vi "Initialize Menus.vi"(8 "Error In":errorcluster, 11 "Menu Controls":refnum<vi>[](array[refnum])) -> (0 "Error Out":errorcluster)   [LabVIEW 2019, in "LMH-LINX.lvlib"]
uses:
  <vilib>/MakerHub/LINX/LMH-LINX.lvlib
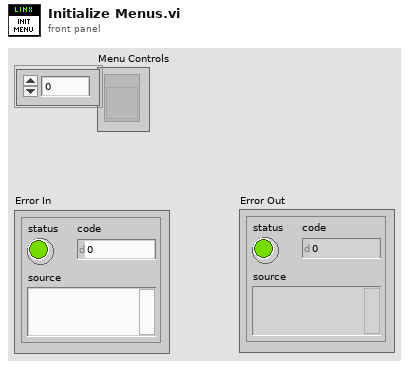
[diagram p1: front panel]
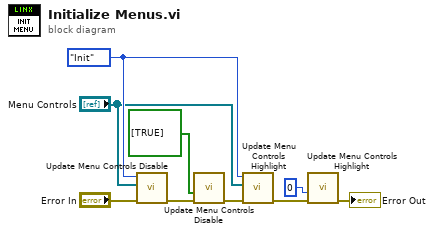
[diagram p0: block diagram]
diagram:
  w6 = enum16{"Init", "Update"}."Init" ("State")
  n1 = call <vilib>:"Update Menu Controls Disable.vi"("Error In"="Error In", "Controls"="Menu Controls", "State"=w6) -> ("Error Out"=w7:errorcluster)  [unwired: 8 in]
  n2 = call <vilib>:"Update Menu Controls Disable.vi"("Error In"=w7, "Enabled?"=bool[] [TRUE]) -> ("Error Out"=w8:errorcluster)  [unwired: 9 in]
  n3 = call <vilib>:"Update Menu Controls Highlight.vi"("Error In"=w8, "Controls"="Menu Controls", "State"=w6) -> ("Error Out"=w2:errorcluster)  [unwired: 8 in]
  n4 = call <vilib>:"Update Menu Controls Highlight.vi"("Error In"=w2, "Selected Index"=0) -> ("Error Out"=→"Error Out":errorcluster)  [unwired: 9 in]
